vi "pmu_Build Trigger Reason.vi"(4 "user defined trigger reason":u8=8 min=8 max=15, 5 "manual":bool, 6 "digital":bool, 7 "magnitude low":bool, 8 "df/dt high":bool, 9 "frequency high/low":bool, 10 "phase-angle diff":bool, 11 "magnitude high":bool) -> (3 "trigger reason":u8 format="%04b")   [LabVIEW 2011, in "NI_EP_PMU.lvlib"]
doc: "This VI encodes trigger reason part of the IEEE C37.118-2005 data message."
uses:
  <vilib>/addons/Electrical Power/PMU/NI_EP_PMU.lvlib
panel:
  # "0111: Digital 0110: Reserved\n0101: df/dt high 0100: Frequency high/low\n0011: Phase-angle diff 0010: Magnitude high\n0001: Magnitude low 0000: Manual"
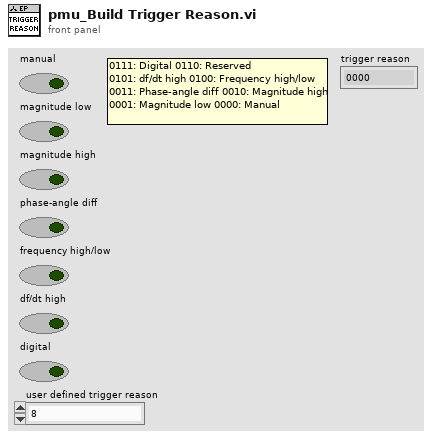
[diagram p1: front panel]
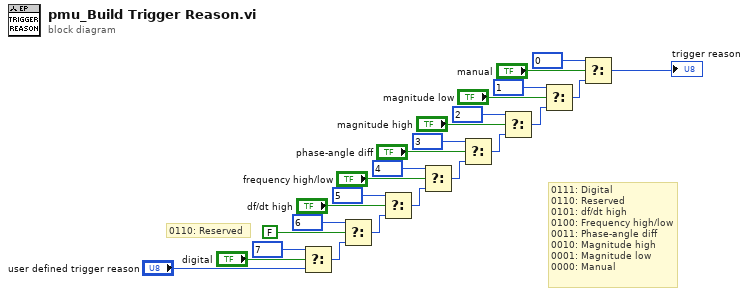
[diagram p0: block diagram]
diagram:
  # "0110: Reserved"
  # "0111: Digital\n0110: Reserved\n0101: df/dt high\n0100: Frequency high/low\n0011: Phase-angle diff\n0010: Magnitude high\n0001: Magnitude low\n0000: Manual"
  n1 = Select(t=u8 7 ("user defined trigger reason 2"), s="digital", f="user defined trigger reason") -> (s? t:f=w3:u8)
  n2 = Select(t=u8 6 ("user defined trigger reason 2"), s=FALSE, f=w3) -> (s? t:f=w4:u8)
  n3 = Select(t=u8 5 ("user defined trigger reason 2"), s="df/dt high", f=w4) -> (s? t:f=w5:u8)
  n4 = Select(t=u8 4 ("user defined trigger reason 2"), s="frequency high/low", f=w5) -> (s? t:f=w6:u8)
  n5 = Select(t=u8 3 ("user defined trigger reason 2"), s="phase-angle diff", f=w6) -> (s? t:f=w7:u8)
  n6 = Select(t=u8 2 ("user defined trigger reason 2"), s="magnitude high", f=w7) -> (s? t:f=w8:u8)
  n7 = Select(t=u8 1 ("user defined trigger reason 2"), s="magnitude low", f=w8) -> (s? t:f=w9:u8)
  n8 = Select(t=u8 0 ("user defined trigger reason 2"), s="manual", f=w9) -> (s? t:f=→"trigger reason":u8)
